vi "Caculate Force.vi"(6 "Arrow Scale":dbl=50.0, 9 "Measured Position":dbl[](array[numeric]), 10 "Robot Force in":dbl[](array[numeric])) -> (1 "Scaled Force":dbl[](array[numeric]), 3 "Performance":dbl, 4 "Robot Force out":dbl[](array[numeric])=[0.27195732694797004, -0.3746074750306182])   [LabVIEW 2021]
uses:
  <vilib>/Analysis/3filter.llb/Filter Passband Type.ctl
  <vilib>/Analysis/BLAS.llb/dnrm2 - Vector 2-Norm (DBL).vi
  <vilib>/Analysis/NI_AALBLAS.lvlib
  <vilib>/ptbypt/NI_PtbyPt.lvlib
  <vilib>/Analysis/NI_AALBase.lvlib
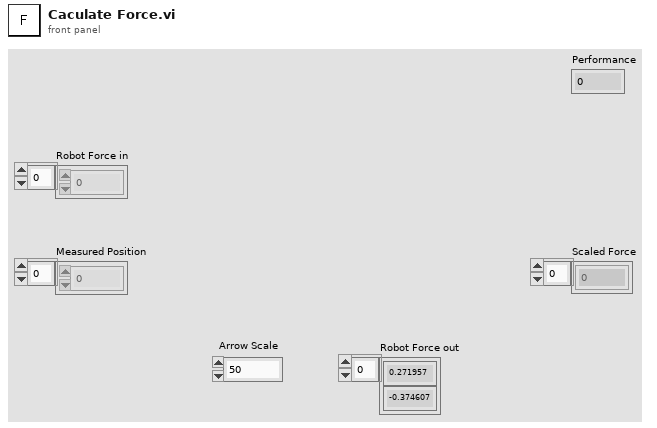
[diagram p1: front panel]
types:
  T1 = typedef "NI_AALBase.lvlib/Filter Passband Type.ctl" = enum32{"Lowpass", "Highpass", "Bandpass", "Bandstop"}
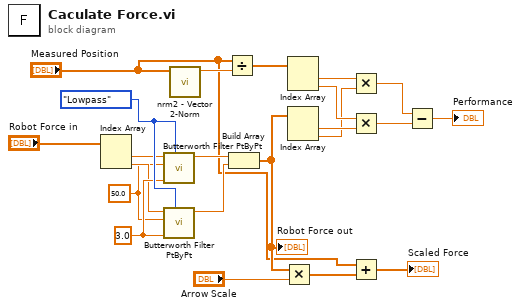
[diagram p0: block diagram]
diagram:
  w14 = Filter_Passband_Type."Lowpass" ("filter type")
  w13 = 3.0 ("low cutoff freq: fl")
  w8 = 50.0 ("sampling freq: fs")
  n1 = Index Array(array="Robot Force in") -> (element #1=w7:dbl, element #2=w9:dbl)  [unwired: 2 in]
  n2 = call <vilib>:"Butterworth Filter PtByPt.vi"("filter type"=w14, "low cutoff freq: fl"=w13, "sampling freq: fs"=w8, "x"=w7) -> ("Filtered x"=w10:dbl)  [unwired: 5 in, 1 out]
  n3 = call <vilib>:"Butterworth Filter PtByPt.vi"("filter type"=w14, "low cutoff freq: fl"=w13, "sampling freq: fs"=w8, "x"=w9) -> ("Filtered x"=w11:dbl)  [unwired: 5 in, 1 out]
  n4 = call-poly <vilib>:"nrm2 - Vector 2-Norm.vi"("x"="Measured Position") -> ("dnrm2"=w3:dbl)  [unwired: 9 in, 1 out]
  n5 = Divide(x="Measured Position", y=w3) -> (x/y=w1:dbl[])
  n6 = Build Array(w10, w11) -> (w15:dbl[])
  "Robot Force out" <- w15
  n7 = Multiply(x=w15, y="Arrow Scale") -> (x*y=w6:dbl[])
  n8 = Index Array(array=w1) -> (element #1=w16:dbl, element #2=w18:dbl)  [unwired: 2 in]
  n9 = Index Array(array=w15) -> (element #1=w19:dbl, element #2=w17:dbl)  [unwired: 2 in]
  n10 = Multiply(x=w16, y=w17) -> (x*y=w20:dbl)
  n11 = Multiply(x=w18, y=w19) -> (x*y=w21:dbl)
  n12 = Add(x="Measured Position", y=w6) -> (x+y=→"Scaled Force":dbl[])
  n13 = Subtract(x=w20, y=w21) -> (x-y=→"Performance":dbl)
